vi "HWCEventHandler.vi"(8 "error in (no error)":errorcluster, 11 "HWController in":refnum<class "HWController.lvclass">) -> (0 "error out":errorcluster, 3 "HWController out":refnum<class "HWController.lvclass">)   [LabVIEW 2011, in "Hardware.lvlib" / "HWControllers.lvlib" / "HWController.lvclass"]
uses:
  HWController.lvclass
  HWController.lvclass/HWController.ctl
  HWControllerEvents/HWControllerEvents.lvclass
panel:
  out "configureTime":dbl
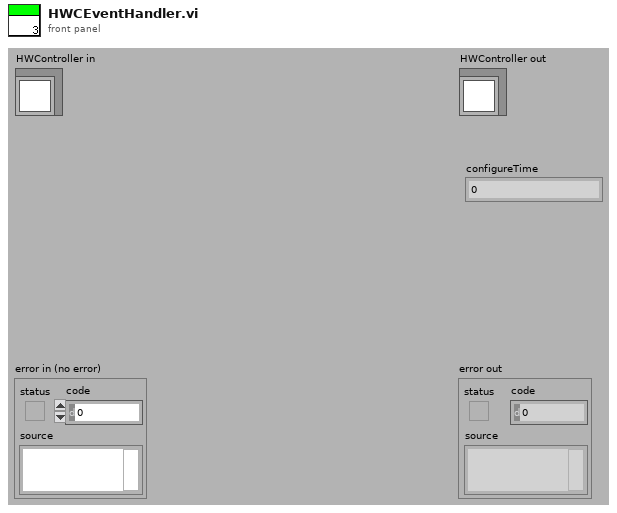
[diagram p1: front panel]
types:
  T1 = enum16{"Ready", "Compiling", "Configured", "Running", "Stopping", "Unresolved Error"}
  T2 = cluster{"incomingEventTypes":cluster{"start":cluster{"Boolean":bool}, "stop":cluster{"Boolean":bool}, "statusInquiry":cluster{"Boolean":bool}, "configure":cluster{"DPScriptPath":path, "TimeStamp":string, "HWLoop?":bool}, "resetError":cluster{"Boolean":bool}, "resourcesInquiry":cluster{"Boolean":bool}, "reserveResources":cluster{"HWList":string[]}, "initialise":cluster{"HWList":string[]}, "close":cluster{"Boolean":bool}, "resetAllChannels":cluster{"Boolean":bool}, "staticChannelUpdate":cluster{"channel_address":string, "calibratedValue":dbl}, "runScript":cluster{"DPScriptPath":path, "TimeStamp":string, "HWLoop?":bool}, "compilingScript":cluster{"Path":path}, "compiledScript":cluster{"Path":path, "timeCompileAt":string}, "compilerError":cluster{"Path":path}, "configureCompiledScript":cluster{"DPScriptPath":path, "TimeStamp":string, "HWLoop?":bool, "CompiledScript":cluster{"ScriptListCompiler.lvclass":refnum<class "ScriptListCompiler.lvclass">, "aoChannels":refnum<class "AnalogOutput.lvclass">[], "doChannels":refnum<class "DigitalOutput.lvclass">[], "rfChannels":refnum<class "DDSOutput.lvclass">[]}}, "restartCompiler":cluster{"restart":bool}, "staticRfChannelUpdate":cluster{"channel_address":string, "Output":cluster{"Frequency(MHz)":dbl, "Amplitude":dbl, "Phase":dbl, "OutputForm":enum16{"Sine", "Square", "Triangle", "Arbitrary"}}}, "cameraUpdate":cluster{"Camera":string, "Type":string, "settings":path}}, "outgoingEventTypes":cluster{"HWStatus":cluster{"status":enum16{"Ready", "Compiling", "Configured", "Running", "Stopping", "Unresolved Error"}}, "error":cluster{"error out":errorcluster}, "resourcesAvailable":cluster{"availableHWList":string[], "reservedHWList":string[]}, "resourcesReserved":cluster{"reservedHWList":string[]}}}
  T3 = enum16{"start", "stop", "statusInquiry", "configure", "resetError", "resourcesInquiry", "reserveResources", "initialise", "resetAllChannels", "staticUpdate", "close", "HWStatus", "error", "resourcesAvailable", "resourcesReserved", "compilerError", "compiledScript", "compilingScript", "runScript", "configureCompiledScript", "restartCompiler", "staticRfChannelUpdate", "cameraUpdate"}
  T4 = cluster{"start":cluster{"Boolean":bool}, "stop":cluster{"Boolean":bool}, "statusInquiry":cluster{"Boolean":bool}, "configure":cluster{"DPScriptPath":path, "TimeStamp":string, "HWLoop?":bool}, "resetError":cluster{"Boolean":bool}, "resourcesInquiry":cluster{"Boolean":bool}, "reserveResources":cluster{"HWList":string[]}, "initialise":cluster{"HWList":string[]}, "close":cluster{"Boolean":bool}, "resetAllChannels":cluster{"Boolean":bool}, "staticChannelUpdate":cluster{"channel_address":string, "calibratedValue":dbl}, "runScript":cluster{"DPScriptPath":path, "TimeStamp":string, "HWLoop?":bool}, "compilingScript":cluster{"Path":path}, "compiledScript":cluster{"Path":path, "timeCompileAt":string}, "compilerError":cluster{"Path":path}, "configureCompiledScript":cluster{"DPScriptPath":path, "TimeStamp":string, "HWLoop?":bool, "CompiledScript":cluster{"ScriptListCompiler.lvclass":refnum<class "ScriptListCompiler.lvclass">, "aoChannels":refnum<class "AnalogOutput.lvclass">[], "doChannels":refnum<class "DigitalOutput.lvclass">[], "rfChannels":refnum<class "DDSOutput.lvclass">[]}}, "restartCompiler":cluster{"restart":bool}, "staticRfChannelUpdate":cluster{"channel_address":string, "Output":cluster{"Frequency(MHz)":dbl, "Amplitude":dbl, "Phase":dbl, "OutputForm":enum16{"Sine", "Square", "Triangle", "Arbitrary"}}}, "cameraUpdate":cluster{"Camera":string, "Type":string, "settings":path}}
  T5 = cluster{"DPScriptPath":path, "TimeStamp":string, "HWLoop?":bool}
  T6 = cluster{"DPScriptPath":path, "TimeStamp":string, "HWLoop?":bool, "CompiledScript":cluster{"ScriptListCompiler.lvclass":refnum<class "ScriptListCompiler.lvclass">, "aoChannels":refnum<class "AnalogOutput.lvclass">[], "doChannels":refnum<class "DigitalOutput.lvclass">[], "rfChannels":refnum<class "DDSOutput.lvclass">[]}}
  T7 = cluster{"ScriptListCompiler.lvclass":refnum<class "ScriptListCompiler.lvclass">, "aoChannels":refnum<class "AnalogOutput.lvclass">[], "doChannels":refnum<class "DigitalOutput.lvclass">[], "rfChannels":refnum<class "DDSOutput.lvclass">[]}
  T8 = cluster{"channel_address":string, "calibratedValue":dbl}
  T9 = cluster{"channel_address":string, "Output":cluster{"Frequency(MHz)":dbl, "Amplitude":dbl, "Phase":dbl, "OutputForm":enum16{"Sine", "Square", "Triangle", "Arbitrary"}}}
  T10 = cluster{"Camera":string, "Type":string, "settings":path}
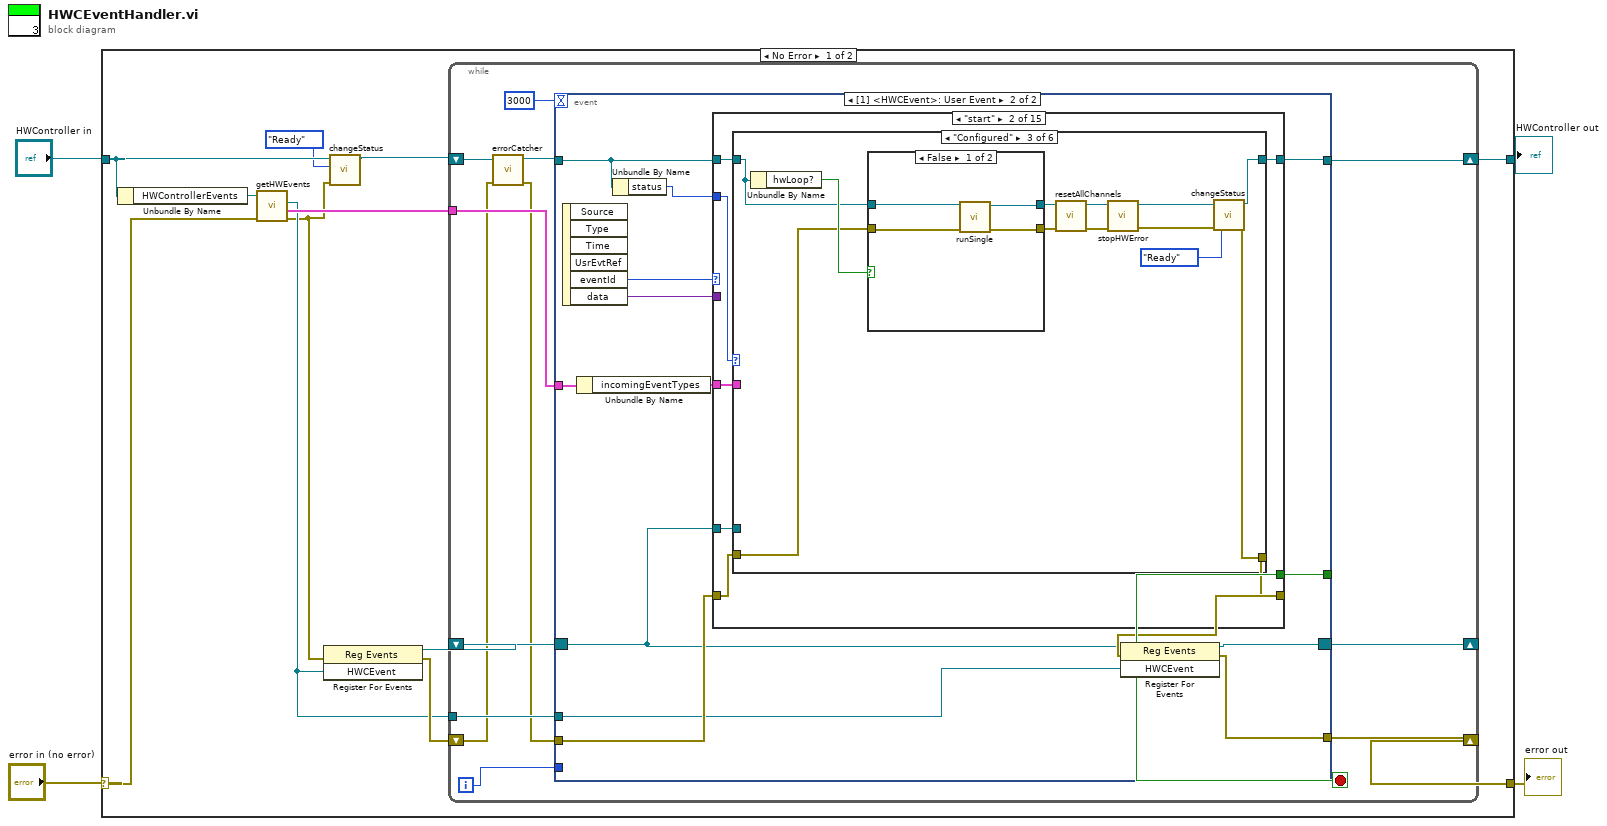
[diagram p0: block diagram]
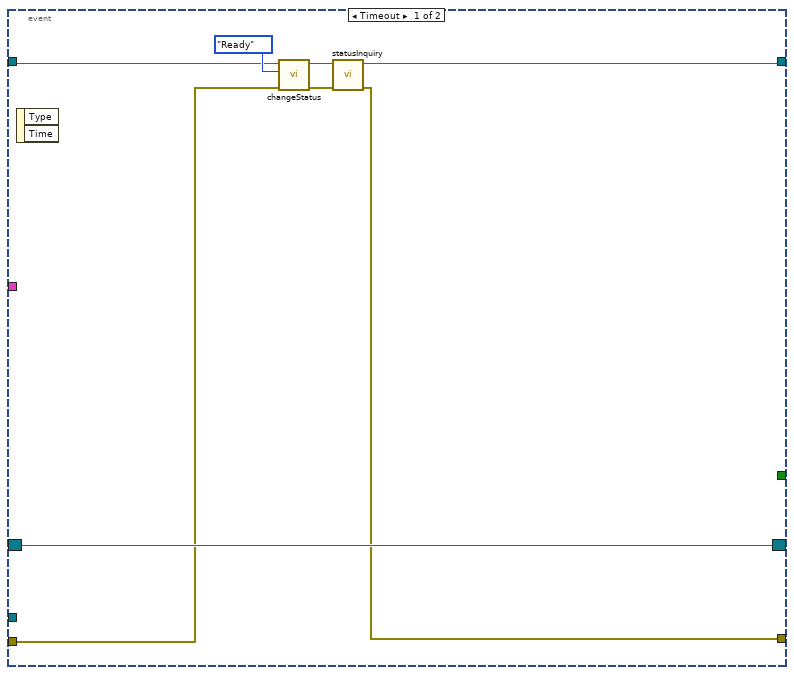
[diagram p2: hidden frame]
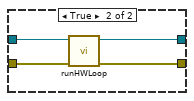
[diagram p6: hidden frame]
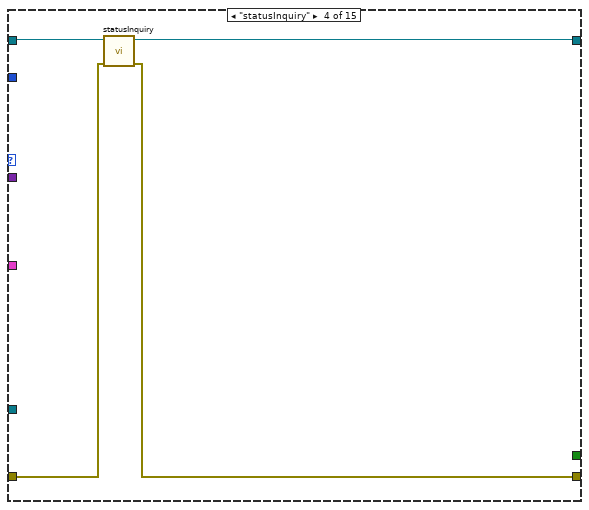
[diagram p11: hidden frame]
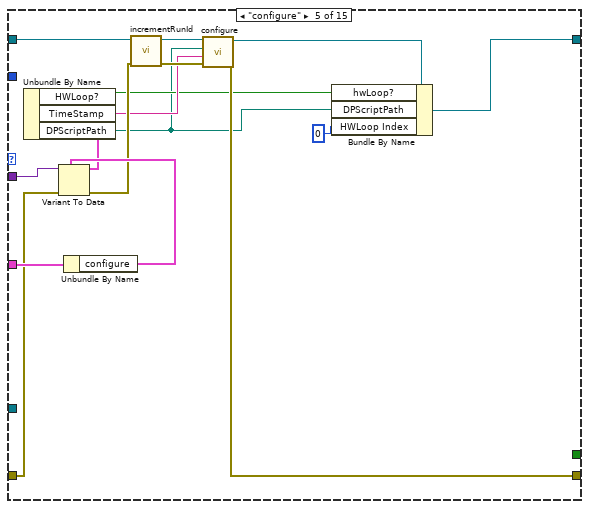
[diagram p12: hidden frame]
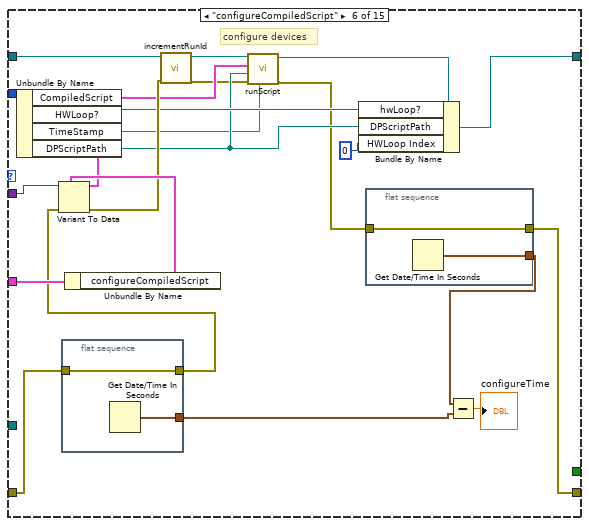
[diagram p13: hidden frame]
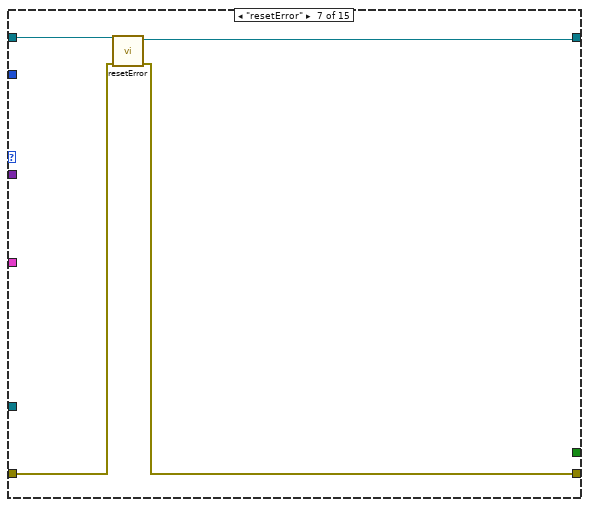
[diagram p14: hidden frame]
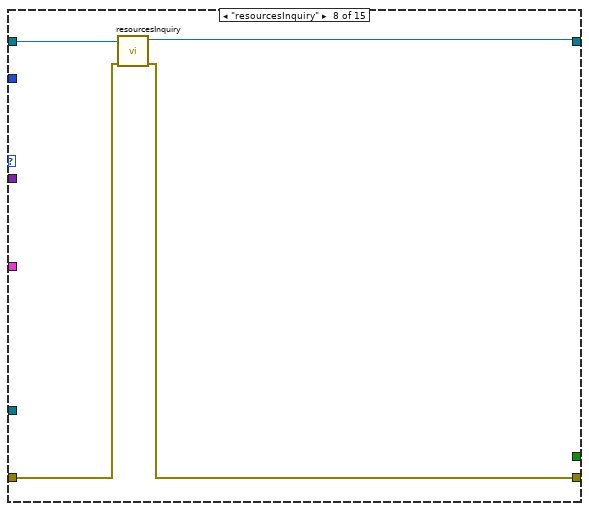
[diagram p15: hidden frame]
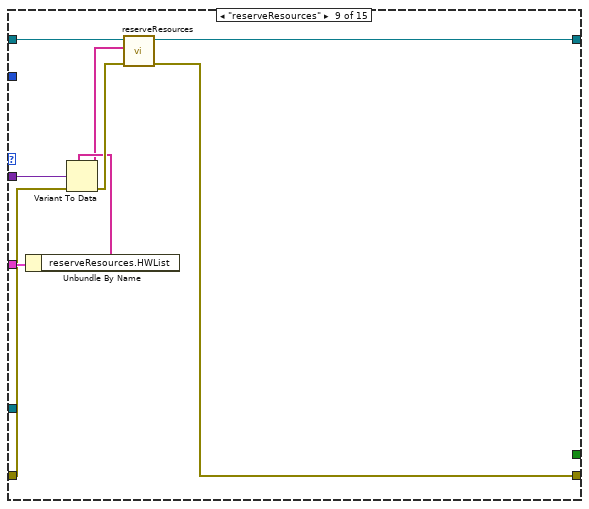
[diagram p16: hidden frame]
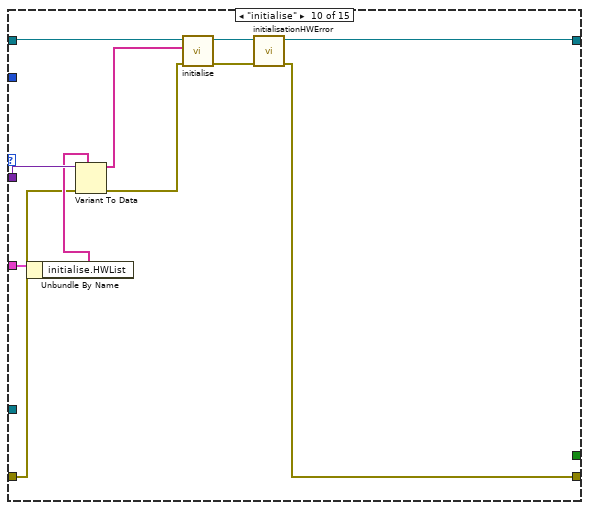
[diagram p17: hidden frame]
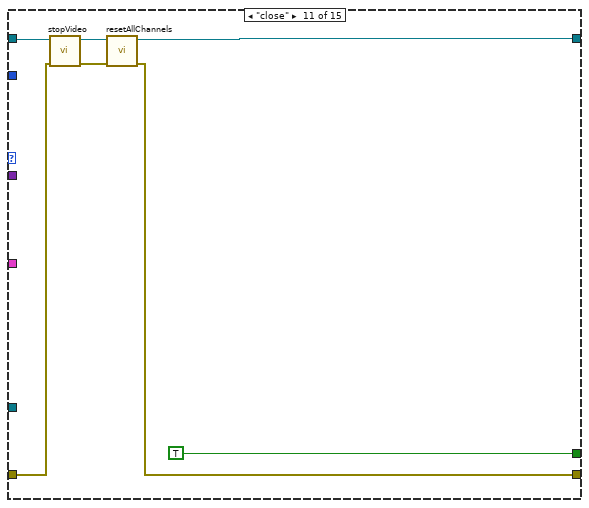
[diagram p18: hidden frame]
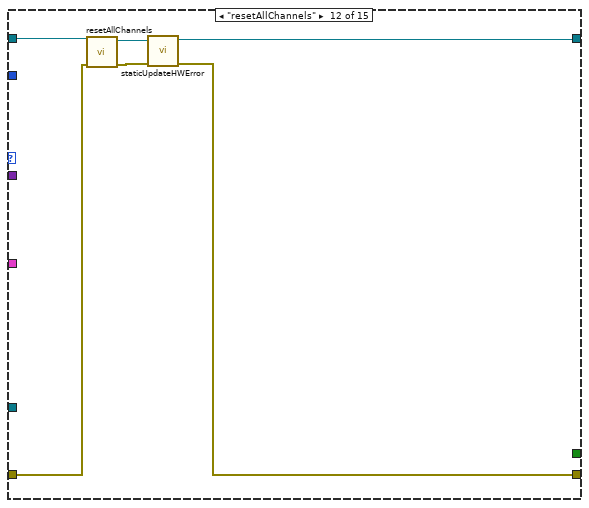
[diagram p19: hidden frame]
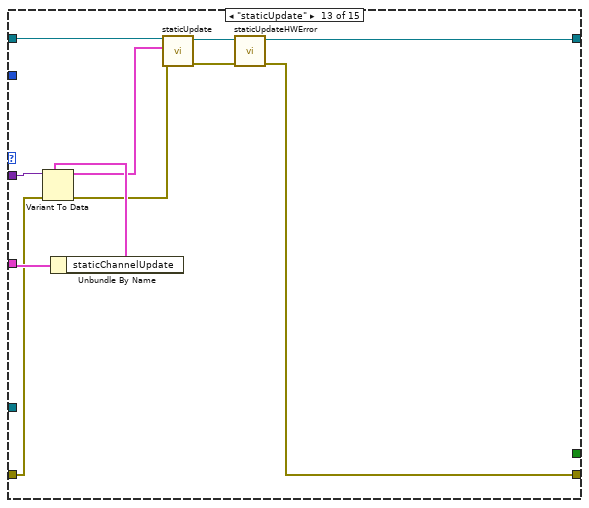
[diagram p20: hidden frame]
diagram:
  n1 = case shown="No Error" "error in (no error)" {
    selector: "error in (no error)" -> [w15 w212]
    tunnel: [w11 w212] -> w3
    tunnel: [w10 w211] -> w1
    tunnel: "HWController in" -> [w8 w211]
    frame No Error {
      n2 = Unbundle By Name(w8) -> ("HWControllerEvents"=w16:refnum<class "HWControllerEvents.lvclass">)
      n3 = call-dynamic "getHWEvents.vi"("error in (no error)"=w15, "HWControllerEvents in"=w16) -> ("error out"=w7:errorcluster, "eventDataTypes"=w12:T2, "HWCEvent"=w9:refnum<user-event>)  [unwired: 6 in, 1 out]
      n4 = register-events(error in=w7, w9) -> (reference out=w13:refnum<event-registration>, error out=w14:errorcluster)  [unwired: 1 in]
      n5 = call "changeStatus.vi"("error in (no error)"=w7, "status"=T1."Ready", "HWController in"=w8) -> ("HWController out"=w5:refnum<class "HWController.lvclass">)  [unwired: 7 in, 1 out]
      n6 = while {
        shift-right: [w29] -> w10
        shift-left: w5 -> [w21]
        shift-right: [w27] -> w11
        shift-left: w14 -> [w20]
        tunnel: w12 -> [w25]
        tunnel: w9 -> [w24]
        shift-right: [w23] -> _
        shift-left: w13 -> [w28]
        i -> [w17]
        stop <- w26 stop-if-true
        n7 = call-dynamic "errorCatcher.vi"("error in (no error)"=w20, "HWController in"=w21) -> ("error out"=w19:errorcluster, "HWController out"=w22:refnum<class "HWController.lvclass">)  [unwired: 8 in]
        n8 = event shown="[1] <HWCEvent>: User Event" {
          selector: w28 -> [w37 w43]
          dyn-events: [w37 w41] -> w23
          timeout: 3000 -> [_ _]
          tunnel: w22 -> [w32 w39]
          tunnel: [w36 w44] -> w29
          tunnel: [w35 w40] -> w27
          tunnel: w19 -> [w30 w50]
          tunnel: [_ w49] -> w26
          tunnel: w25 -> [_ w48]
          tunnel: w24 -> [_ w42]
          tunnel: w17 -> [_ _]
          event Timeout {
            n9 = event-data() -> ()  [unwired: 1 in, 2 out]
            n10 = call "changeStatus.vi"("error in (no error)"=w30, "status"=T1."Ready", "HWController in"=w32) -> ("error out"=w31:errorcluster, "HWController out"=w33:refnum<class "HWController.lvclass">)  [unwired: 7 in]
            n11 = call-dynamic "statusInquiry.vi"("error in (no error)"=w31, "HWController in"=w33) -> ("error out"=w35:errorcluster, "HWController out"=w36:refnum<class "HWController.lvclass">)  [unwired: 8 in]
          }
          event User Event {
            n12 = event-data() -> ("eventId"=w51:T3, "data"=w46:variant)  [unwired: 1 in, 4 out]
            n13 = Unbundle By Name(w48) -> ("incomingEventTypes"=w47:T4)
            n14 = Unbundle By Name(w39) -> ("status"=w38:T1)
            n15 = case shown="\"start\"" w51 {
              tunnel: w39 -> [w53 w60 w92 w96 w106 w113 w142 w146 w154 w165 w170 w179 w190 w197 w206]
              tunnel: [w53 w58 w92 w95 w98 w128 w141 w145 w153 w156 w172 w175 w181 w191 w205] -> w44
              tunnel: w50 -> [w52 w56 w91 w94 w109 w120 w140 w144 w150 w161 w167 w178 w185 w198 w207]
              tunnel: [w52 w57 w91 w93 w107 w117 w139 w143 w152 w157 w171 w174 w180 w192 w202] -> w45
              tunnel: [_ _ _ _ _ _ _ _ _ _ TRUE _ _ _ _] -> w49
              tunnel: w47 -> [_ w54 _ _ w112 w134 _ _ w155 w166 _ _ w188 w200 w209]
              tunnel: w46 -> [_ _ _ _ w110 w132 _ _ w151 w164 _ _ w189 w201 w210]
              tunnel: w43 -> [_ w59 _ _ _ _ _ _ _ _ _ _ _ _ _]
              tunnel: w38 -> [_ w55 _ _ _ _ _ _ _ _ _ _ _ _ _]
              frame Default {
                # "Do not respond to outgoing events."
              }
              frame "start" {
                n16 = case shown="\"Configured\"" w55 {
                  tunnel: w60 -> [w62 w64 w73 w86 w88 w90]
                  tunnel: w59 -> [_ _ _ _ _ _]
                  tunnel: [w62 w64 w67 w86 w88 w90] -> w58
                  tunnel: [w61 w63 w69 w85 w87 w89] -> w57
                  tunnel: w56 -> [w61 w63 w70 w85 w87 w89]
                  tunnel: w54 -> [_ _ _ _ _ _]
                  frame "Ready", Default {
                  }
                  frame "Compiling" {
                  }
                  frame "Configured" {
                    n17 = Unbundle By Name(w73) -> ("hwLoop?"=w76:bool)
                    n18 = case shown="False" w76 {
                      tunnel: w70 -> [w79 w81]
                      tunnel: [w78 w83] -> w75
                      tunnel: [w77 w82] -> w74
                      tunnel: w73 -> [w80 w84]
                      frame False {
                        n19 = call "runSingle.vi"("error in (no error)"=w79, "HWController in"=w80) -> ("error out"=w77:errorcluster, "HWController out"=w78:refnum<class "HWController.lvclass">)  [unwired: 6 in, 2 out]
                      }
                      frame True {
                        n20 = call "runHWLoop.vi"("error in (no error)"=w81, "HWController in"=w84) -> ("error out"=w82:errorcluster, "HWController out"=w83:refnum<class "HWController.lvclass">)  [unwired: 8 in]
                      }
                    }
                    n21 = call-dynamic "resetAllChannels.vi"("error in (no error)"=w74, "HWController in"=w75) -> ("error out"=w71:errorcluster, "HWController out"=w72:refnum<class "HWController.lvclass">)  [unwired: 8 in]
                    n22 = call-dynamic "stopHWError.vi"("error in (no error)"=w71, "HWController in"=w72) -> ("error out"=w65:errorcluster, "HWController out"=w66:refnum<class "HWController.lvclass">)  [unwired: 8 in]
                    n23 = call "changeStatus.vi"("error in (no error)"=w65, "status"=T1."Ready", "HWController in"=w66) -> ("error out"=w69:errorcluster, "HWController out"=w67:refnum<class "HWController.lvclass">)  [unwired: 7 in]
                  }
                  frame "Running" {
                  }
                  frame "Stopping" {
                  }
                  frame "Unresolved Error" {
                  }
                }
              }
              frame "stop" {
              }
              frame "statusInquiry" {
                n24 = call-dynamic "statusInquiry.vi"("error in (no error)"=w94, "HWController in"=w96) -> ("error out"=w93:errorcluster, "HWController out"=w95:refnum<class "HWController.lvclass">)  [unwired: 8 in]
              }
              frame "configure" {
                n25 = Unbundle By Name(w112) -> ("configure"=w111:T5)
                n26 = Variant To Data(error in=w109, type=w111, Variant=w110) -> (data=w108:T5, error out=w104:errorcluster)
                n27 = Unbundle By Name(w108) -> ("HWLoop?"=w101:bool, "TimeStamp"=w102:string, "DPScriptPath"=w99:path)
                n28 = call "incrementRunId.vi"("error in (no error)"=w104, "HWController in"=w106) -> ("error out"=w103:errorcluster, "HWController out"=w105:refnum<class "HWController.lvclass">)  [unwired: 8 in]
                n29 = call-dynamic "configure.vi"("error in (no error)"=w103, "timeStamp"=w102, "Path"=w99, "HWController in"=w105) -> ("error out"=w107:errorcluster, "HWController out"=w100:refnum<class "HWController.lvclass">)  [unwired: 6 in]
                n30 = Bundle By Name(cluster=w100, "hwLoop?"=w101, "DPScriptPath"=w99, "HWLoop Index"=0) -> (w98:refnum<class "HWController.lvclass">)
              }
              frame "configureCompiledScript" {
                # "configure devices"
                n31 = flat-sequence {
                  tunnel: w120 -> [w138]
                  tunnel: [w138] -> w119
                  tunnel: [w137] -> w116
                  frame #0 {
                    n32 = Get Date/Time In Seconds() -> (seconds since 1Jan1904=w137:timestamp)
                  }
                }
                n33 = Unbundle By Name(w134) -> ("configureCompiledScript"=w133:T6)
                n34 = Variant To Data(error in=w119, type=w133, Variant=w132) -> (data=w131:T6, error out=w130:errorcluster)
                n35 = Unbundle By Name(w131) -> ("CompiledScript"=w125:T7, "HWLoop?"=w129:bool, "TimeStamp"=w123:string, "DPScriptPath"=w124:path)
                n36 = call "incrementRunId.vi"("error in (no error)"=w130, "HWController in"=w113) -> ("error out"=w122:errorcluster, "HWController out"=w126:refnum<class "HWController.lvclass">)  [unwired: 8 in]
                n37 = call-dynamic "runScript.vi"("timeStamp"=w123, "error in (no error)"=w122, "Path"=w124, "CompiledScript"=w125, "HWController in"=w126) -> ("error out"=w118:errorcluster, "HWController out"=w121:refnum<class "HWController.lvclass">)  [unwired: 5 in]
                n38 = Bundle By Name(cluster=w121, "hwLoop?"=w129, "DPScriptPath"=w124, "HWLoop Index"=0) -> (w128:refnum<class "HWController.lvclass">)
                n39 = flat-sequence {
                  tunnel: w118 -> [w136]
                  tunnel: [w136] -> w117
                  tunnel: [w135] -> w115
                  frame #0 {
                    n40 = Get Date/Time In Seconds() -> (seconds since 1Jan1904=w135:timestamp)
                  }
                }
                n41 = Subtract(x=w115, y=w116) -> (x-y=→"configureTime":dbl)
              }
              frame "resetError" {
                n42 = call-dynamic "resetError.vi"("error in (no error)"=w140, "HWController in"=w142) -> ("error out"=w139:errorcluster, "HWController out"=w141:refnum<class "HWController.lvclass">)  [unwired: 8 in]
              }
              frame "resourcesInquiry" {
                n43 = call-dynamic "resourcesInquiry.vi"("error in (no error)"=w144, "HWController in"=w146) -> ("error out"=w143:errorcluster, "HWController out"=w145:refnum<class "HWController.lvclass">)  [unwired: 8 in]
              }
              frame "reserveResources" {
                n44 = Unbundle By Name(w155) -> ("reserveResources.HWList"=w148:string[])
                n45 = Variant To Data(error in=w150, type=w148, Variant=w151) -> (data=w147:string[], error out=w149:errorcluster)
                n46 = call-dynamic "reserveResources.vi"("error in (no error)"=w149, "HWList"=w147, "HWController in"=w154) -> ("error out"=w152:errorcluster, "HWController out"=w153:refnum<class "HWController.lvclass">)  [unwired: 7 in]
              }
              frame "initialise" {
                n47 = Unbundle By Name(w166) -> ("initialise.HWList"=w163:string[])
                n48 = Variant To Data(error in=w161, type=w163, Variant=w164) -> (data=w162:string[], error out=w160:errorcluster)
                n49 = call-dynamic "initialise.vi"("error in (no error)"=w160, "HWList"=w162, "HWController in"=w165) -> ("error out"=w158:errorcluster, "HWController out"=w159:refnum<class "HWController.lvclass">)  [unwired: 7 in]
                n50 = call-dynamic "initialisationHWError.vi"("error in (no error)"=w158, "HWController in"=w159) -> ("error out"=w157:errorcluster, "HWController out"=w156:refnum<class "HWController.lvclass">)  [unwired: 8 in]
              }
              frame "close" {
                n51 = call-dynamic "stopVideo.vi"("error in (no error)"=w167, "HWController in"=w170) -> ("error out"=w168:errorcluster, "HWController out"=w169:refnum<class "HWController.lvclass">)  [unwired: 8 in]
                n52 = call-dynamic "resetAllChannels.vi"("error in (no error)"=w168, "HWController in"=w169) -> ("error out"=w171:errorcluster, "HWController out"=w172:refnum<class "HWController.lvclass">)  [unwired: 8 in]
              }
              frame "resetAllChannels" {
                n53 = call-dynamic "resetAllChannels.vi"("error in (no error)"=w178, "HWController in"=w179) -> ("error out"=w176:errorcluster, "HWController out"=w177:refnum<class "HWController.lvclass">)  [unwired: 8 in]
                n54 = call-dynamic "staticUpdateHWError.vi"("error in (no error)"=w176, "HWController in"=w177) -> ("error out"=w174:errorcluster, "HWController out"=w175:refnum<class "HWController.lvclass">)  [unwired: 8 in]
              }
              frame "staticUpdate" {
                n55 = Unbundle By Name(w188) -> ("staticChannelUpdate"=w187:T8)
                n56 = Variant To Data(error in=w185, type=w187, Variant=w189) -> (data=w186:T8, error out=w184:errorcluster)
                n57 = call-dynamic "staticUpdate.vi"("error in (no error)"=w184, "staticChannelUpdate"=w186, "HWController in"=w190) -> ("error out"=w182:errorcluster, "HWController out"=w183:refnum<class "HWController.lvclass">)  [unwired: 7 in]
                n58 = call-dynamic "staticUpdateHWError.vi"("error in (no error)"=w182, "HWController in"=w183) -> ("error out"=w180:errorcluster, "HWController out"=w181:refnum<class "HWController.lvclass">)  [unwired: 8 in]
              }
              frame "staticRfChannelUpdate" {
                n59 = Unbundle By Name(w200) -> ("staticRfChannelUpdate"=w199:T9)
                n60 = Variant To Data(error in=w198, type=w199, Variant=w201) -> (data=w196:T9, error out=w195:errorcluster)
                n61 = call-dynamic "staticRFChannelUpdate.vi"("error in (no error)"=w195, "staticChannelUpdate"=w196, "HWController in"=w197) -> ("error out"=w193:errorcluster, "HWController out"=w194:refnum<class "HWController.lvclass">)  [unwired: 7 in]
                n62 = call-dynamic "staticUpdateHWError.vi"("error in (no error)"=w193, "HWController in"=w194) -> ("error out"=w192:errorcluster, "HWController out"=w191:refnum<class "HWController.lvclass">)  [unwired: 8 in]
              }
              frame "cameraUpdate" {
                n63 = Unbundle By Name(w209) -> ("cameraUpdate"=w208:T10)
                n64 = Variant To Data(error in=w207, type=w208, Variant=w210) -> (data=w204:T10, error out=w203:errorcluster)
                n65 = call-dynamic "updateCamera.vi"("error in (no error)"=w203, "data"=w204, "HWController in"=w206) -> ("error out"=w202:errorcluster, "HWController out"=w205:refnum<class "HWController.lvclass">)  [unwired: 7 in]
              }
            }
            n66 = register-events(reference=w43, error in=w45, w42) -> (reference out=w41:refnum<event-registration>, error out=w40:errorcluster)
          }
        }
      }
    }
    frame Error {
    }
  }
  "error out" <- w3
  "HWController out" <- w1
